vi "Grab Frame.vi"(8 "error in (no error)":errorcluster, 9 "Image Refnum":refnum<vi>, 10 "Images":T1[](array[typedef]), 11 "Notifiers":T2) -> (0 "error out":errorcluster, 2 "Image Out":T1)   [LabVIEW 2014]
uses:
  support/Notifiers/Notifiers.ctl
  support/Message Handler Loop Notifiers.ctl
  Parameter Analyzer/Parameter Analyzer Notifiers.ctl
  Switching Matrix/Switching Matrix Notifiers.ctl
  Stress Control/StressControl Notifiers.ctl
  Spectrometer/Spectrometer Notifiers.ctl
  Switches and Mirrors/SwitchesMirrors Notifiers.ctl
  Camera/Camera Notifiers.ctl
  XYZ Stage/XYZ Notifications.ctl
  Autofocus Notifiers.ctl
  Measurements/Optoelectronic Measurement/Optoelectronic Notifiers.ctl
  Measurements/Save Data/SaveData Notifiers.ctl
  Measurements/Instrument Sequence/Instrument Sequence Notifiers.ctl
  <vilib>/vision/Image Controls.llb/IMAQ Image.ctl
  <vilib>/vision/NI_Vision_Development_Module.lvlib
panel:
  # "LICENSED MATERIALS – PROPERTY OF IBM\nCopyright IBM Corp. 2016,\nALL RIGHTS RESERVED"
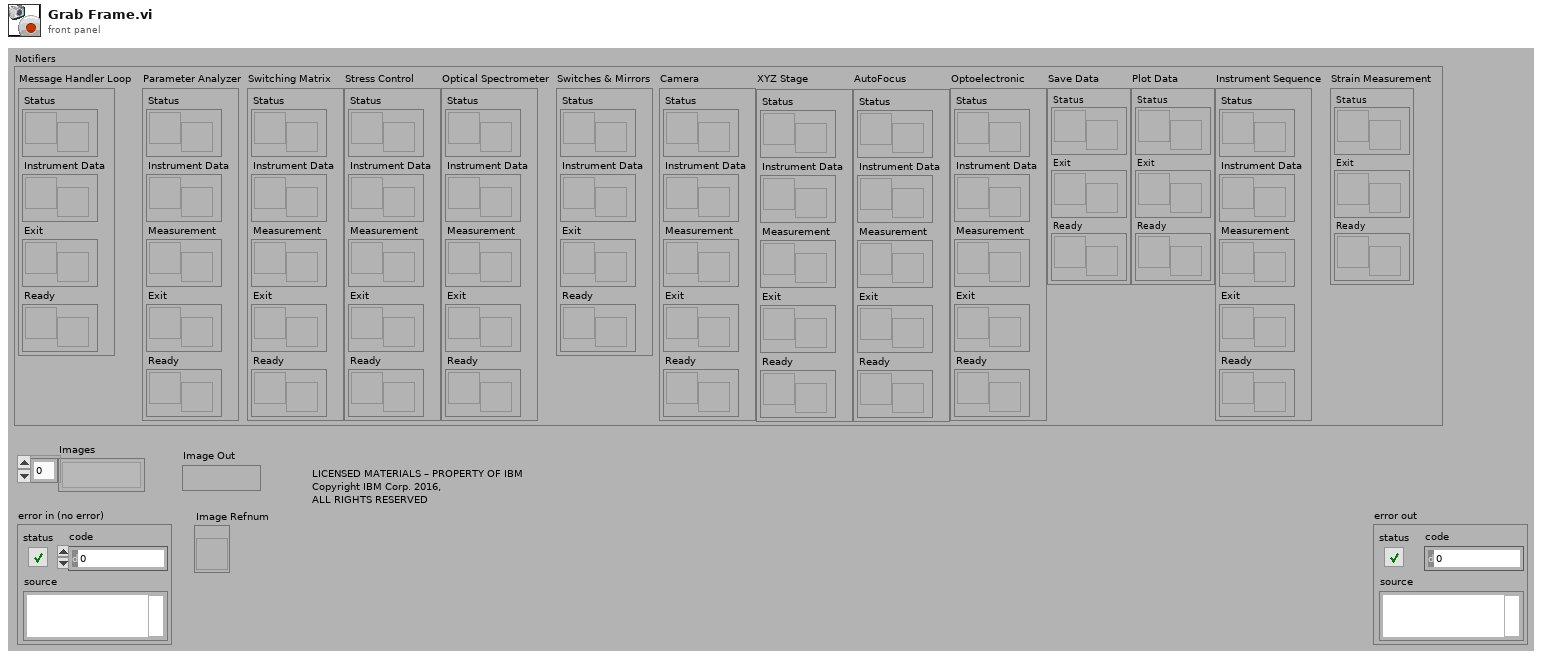
[diagram p1: front panel]
types:
  T1 = typedef "IMAQ Image.ctl" = refnum<image>
  T2 = typedef "Notifiers.ctl" = cluster{"Message Handler Loop":T3, "Parameter Analyzer":T4, "Switching Matrix":T5, "Stress Control":T6, "Optical Spectrometer":T7, "Switches & Mirrors":T8, "Camera":T9, "XYZ Stage":T10, "AutoFocus":T11, "Optoelectronic":T12, "Save Data":T13, "Plot Data":T13, "Instrument Sequence":T14, "Strain Measurement":cluster{"Status":refnum<notifier>, "Exit":refnum<notifier>, "Ready":refnum<notifier>}}
  T3 = typedef "Message Handler Loop Notifiers.ctl" = cluster{"Status":refnum<notifier>, "Instrument Data":refnum<notifier>, "Exit":refnum<notifier>, "Ready":refnum<notifier>}
  T4 = typedef "Parameter Analyzer Notifiers.ctl" = cluster{"Status":refnum<notifier>, "Instrument Data":refnum<notifier>, "Measurement":refnum<notifier>, "Exit":refnum<notifier>, "Ready":refnum<notifier>}
  T5 = typedef "Switching Matrix Notifiers.ctl" = cluster{"Status":refnum<notifier>, "Instrument Data":refnum<notifier>, "Measurement":refnum<notifier>, "Exit":refnum<notifier>, "Ready":refnum<notifier>}
  T6 = typedef "StressControl Notifiers.ctl" = cluster{"Status":refnum<notifier>, "Instrument Data":refnum<notifier>, "Measurement":refnum<notifier>, "Exit":refnum<notifier>, "Ready":refnum<notifier>}
  T7 = typedef "Spectrometer Notifiers.ctl" = cluster{"Status":refnum<notifier>, "Instrument Data":refnum<notifier>, "Measurement":refnum<notifier>, "Exit":refnum<notifier>, "Ready":refnum<notifier>}
  T8 = typedef "SwitchesMirrors Notifiers.ctl" = cluster{"Status":refnum<notifier>, "Instrument Data":refnum<notifier>, "Exit":refnum<notifier>, "Ready":refnum<notifier>}
  T9 = typedef "Camera Notifiers.ctl" = cluster{"Status":refnum<notifier>, "Instrument Data":refnum<notifier>, "Measurement":refnum<notifier>, "Exit":refnum<notifier>, "Ready":refnum<notifier>}
  T10 = typedef "XYZ Notifications.ctl" = cluster{"Status":refnum<notifier>, "Instrument Data":refnum<notifier>, "Measurement":refnum<notifier>, "Exit":refnum<notifier>, "Ready":refnum<notifier>}
  T11 = typedef "Autofocus Notifiers.ctl" = cluster{"Status":refnum<notifier>, "Instrument Data":refnum<notifier>, "Measurement":refnum<notifier>, "Exit":refnum<notifier>, "Ready":refnum<notifier>}
  T12 = typedef "Optoelectronic Notifiers.ctl" = cluster{"Status":refnum<notifier>, "Instrument Data":refnum<notifier>, "Measurement":refnum<notifier>, "Exit":refnum<notifier>, "Ready":refnum<notifier>}
  T13 = typedef "SaveData Notifiers.ctl" = cluster{"Status":refnum<notifier>, "Exit":refnum<notifier>, "Ready":refnum<notifier>}
  T14 = typedef "Instrument Sequence Notifiers.ctl" = cluster{"Status":refnum<notifier>, "Instrument Data":refnum<notifier>, "Measurement":refnum<notifier>, "Exit":refnum<notifier>, "Ready":refnum<notifier>}
  T15 = typedef "Image Type" = u32
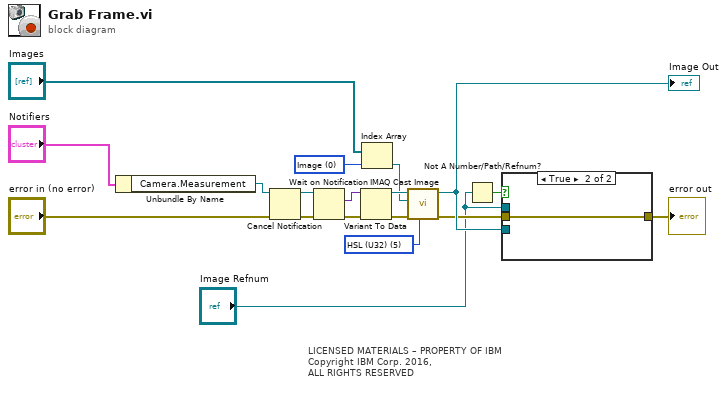
[diagram p0: block diagram]
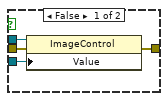
[diagram p2: hidden frame]
diagram:
  w14 = T15 5 items=["Grayscale (U8)", "Grayscale (I16)", "Grayscale (SGL)", "Complex (CSG)", "RGB (U32)", "HSL (U32)", "RGB (U64)", "Grayscale (U16)"] ("Image Type")
  w12 = u16 0 items=["Image", "Template", "Edge"] ("Image Names")
  # "LICENSED MATERIALS – PROPERTY OF IBM\nCopyright IBM Corp. 2016,\nALL RIGHTS RESERVED"
  n1 = Unbundle By Name("Notifiers") -> ("Camera.Measurement"=w9:refnum<notifier>)
  n2 = Cancel Notification(0:w9, 3:"error in (no error)") -> (8:w10:refnum<notifier>, 11:w7:errorcluster)  [unwired: 1 out]
  n3 = Wait on Notification(notifier=w10, error in (no error)=w7) -> (notification=w11:variant, error out=w8:errorcluster)  [unwired: 2 in, 2 out]
  n4 = Variant To Data(error in=w8, Variant=w11) -> (data=w16:T1, error out=w15:errorcluster)  [unwired: 1 in]
  n5 = Index Array(array="Images", index=w12) -> (element=w13:T1)
  n6 = call "IMAQ Cast Image"("Image Type"=w14, "error in (no error)"=w15, "Image Dst"=w13, "Image Src"=w16) -> ("error out"=w4:errorcluster, "Image Dst Out"=w5:T1)  [unwired: 2 in, 4 out]
  "Image Out" <- w5
  n7 = Not A Number/Path/Refnum?(number/path/refnum="Image Refnum") -> (NaN/Path/Refnum?=w2:bool)
  n8 = case shown="True" w2 {
    tunnel: "Image Refnum" -> [w22 _]
    tunnel: w5 -> [w21 _]
    tunnel: w4 -> [w20 w23]
    tunnel: [w19 w23] -> w3
    frame False {
      n9 = property class="ImageControl"(reference=w22, error in=w20, "Value"=w21) -> (error out=w19:errorcluster)  [unwired: 1 out]
    }
    frame True {
    }
  }
  "error out" <- w3
